vi "start_sweep.vi"(8 "error in (no error)":errorcluster, 11 "ScanModeDL091001Scaffold in":refnum<class "ImagingModeDL100901FlexTrajectory.lvclass">) -> (0 "error out":errorcluster, 3 "ScanModeDL091001Scaffold out":refnum<class "ImagingModeDL100901FlexTrajectory.lvclass">)   [LabVIEW 2010, in "ImagingModeDL100901FlexTrajectory.lvclass"]
uses:
  ImagingModeDL100901FlexTrajectory.lvclass
  ImagingModeDL100901FlexTrajectory.lvclass/ImagingModeDL100901FlexTrajectory.ctl
  ImagingModeDL091001Scaffold/ImagingModeDL091001Scaffold/ImagingModeDL091001Scaffold.lvclass
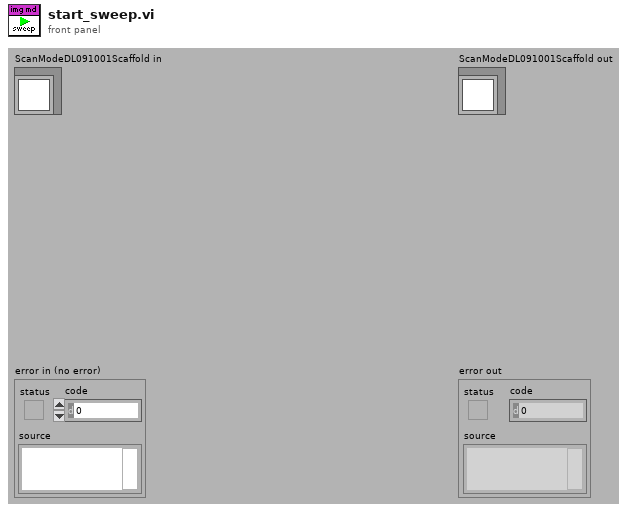
[diagram p1: front panel]
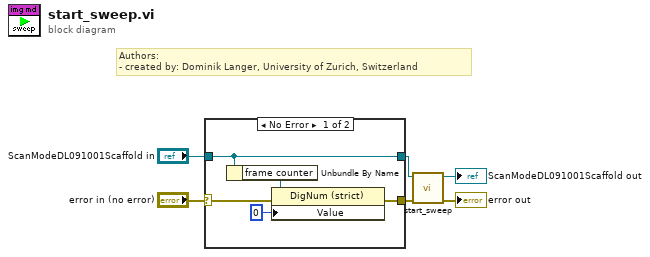
[diagram p0: block diagram]
diagram:
  # "Authors: \n- created by: Dominik Langer, University of Zurich, Switzerland"
  n1 = case shown="No Error" "error in (no error)" {
    selector: "error in (no error)" -> [w9 w12]
    tunnel: [w8 w12] -> w3
    tunnel: "ScanModeDL091001Scaffold in" -> [w11 w13]
    tunnel: [w11 w13] -> w1
    frame No Error {
      n2 = Unbundle By Name(w11) -> ("frame counter"=w10:refnum<vi>)
      n3 = property class="DigNum (strict)"(reference=w10, error in=w9, "Value"=0) -> (error out=w8:errorcluster)  [unwired: 1 out]
    }
    frame Error {
    }
  }
  n4 = call-parent "start_sweep.vi"("error in (no error)"=w3, "ScanModeDL091001Scaffold in"=w1) -> ("error out"=→"error out":errorcluster, "ScanModeDL091001Scaffold out"=→"ScanModeDL091001Scaffold out":refnum<class "ImagingModeDL100901FlexTrajectory.lvclass">)  [unwired: 8 in]
